vi "status of worker4.vi"() -> ()   [LabVIEW 2020]
panel:
  out "worker4_busy/ready":bool
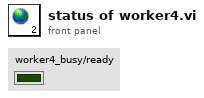
[diagram p1: front panel]
diagram:
